vi "RotateToDegrees.vi"(9 "Trigger Range":dbl=12.0, 11 "Angle Setpoint":dbl=-50.0 format="%#_13g") -> (0 "Triggered":bool, 2 "Right Motor Value":dbl=-1.0, 3 "Left Motor Value":dbl=1.0)   [LabVIEW 2018]
uses:
  <vilib>/addons/control/pid/pid.llb/PID (DBL).vi
  <vilib>/Rock Robotics/WPI/Joystick/WPI_JoystickArcadeMapping.vi
  <vilib>/addons/control/pid/NI_PID_pid.lvlib
panel:
  in  "PID gains 2":T1={"proportional gain (Kc)"=0.04900000000000001, "integral time (Ti, min)"=0.0, "derivative time (Td, min)"=0.002} {"derivative time (Td, min)" format="%.3f"; "integral time (Ti, min)" format="%.3f"; "proportional gain (Kc)" format="%.3f"}
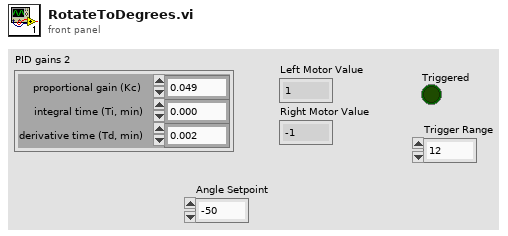
[diagram p1: front panel]
types:
  T1 = cluster{"proportional gain (Kc)":dbl, "integral time (Ti, min)":dbl, "derivative time (Td, min)":dbl}
  T2 = enum16{"[0, 360]", "[-180, 180]", "[0, 2PI]", "[-PI, PI]"}
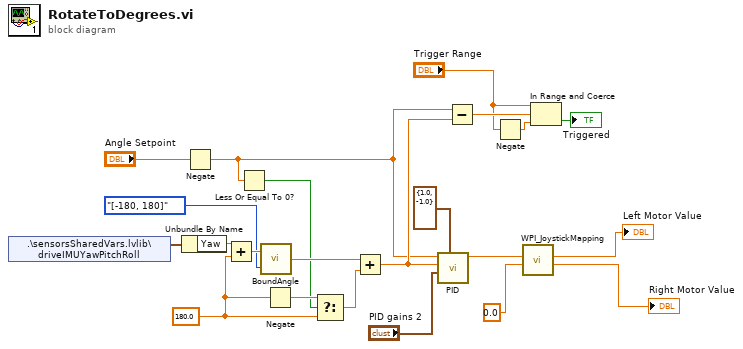
[diagram p0: block diagram]
diagram:
  w11 = 180.0 ("y")
  n1 = shared-variable ".\\sensorsSharedVars.lvlib\\driveIMUYawPitchRoll"() -> (w22:cluster{"Yaw":dbl, "Pitch":dbl, "Roll":dbl})  [unwired: 1 in, 1 out]
  n2 = Unbundle By Name(w22) -> ("Yaw"=w18:dbl)
  n3 = Negate(x="Angle Setpoint") -> (-x=w5:dbl)
  n4 = Add(x=w18, y=w11) -> (x+y=w17:dbl)
  n5 = Less Or Equal To 0?(x=w5) -> (x <= 0?=w9:bool)
  n6 = call <userlib>:"BoundAngle.vi"("Type"=T2."[-180, 180]", "Angle"=w17) -> ("Bound Angle"=w15:dbl)
  n7 = Negate(x=w11) -> (-x=w12:dbl)
  n8 = Select(t=w12, s=w9, f=w11) -> (s? t:f=w13:dbl)
  n9 = Add(x=w15, y=w13) -> (x+y=w6:dbl)
  n10 = call-poly <vilib>:"PID.vi"("output range"=cluster{"output high":dbl, "output low":dbl} {"output high"=1.0, "output low"=-1.0}, "PID gains"="PID gains 2", "process variable"=w6, "setpoint"=w5) -> ("output"=w14:dbl)  [unwired: 6 in, 1 out]
  n11 = Subtract(x=w5, y=w6) -> (x-y=w4:dbl)
  n12 = Negate(x="Trigger Range") -> (-x=w3:dbl)
  n13 = call-poly <vilib>:"WPI_JoystickMapping.vi"("Y axis value"=0.0, "X axis value"=w14) -> ("Right Motor Value"=→"Right Motor Value":dbl, "Left Motor Value"=→"Left Motor Value":dbl)  [unwired: 8 in]
  n14 = In Range and Coerce(upper limit="Trigger Range", x=w4, lower limit=w3) -> (In Range?=→"Triggered":bool)  [unwired: 1 out]
